vi "Add Modifier to File Name.vi"(1 "file name modifier":string, 2 "base path":path) -> (0 "appended path":path)   [LabVIEW 2021, in "Logging.lvlib"]
doc: "Take 'base path' and append 'file name modifier' to the name part of the path, keeping the same exension. Returned in 'appended path'."
uses:
  Logging.lvlib
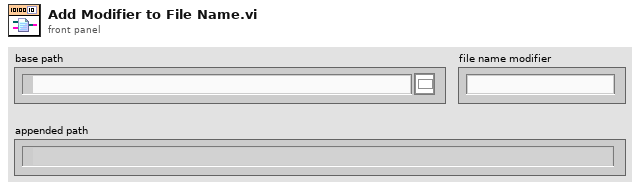
[diagram p1: front panel]
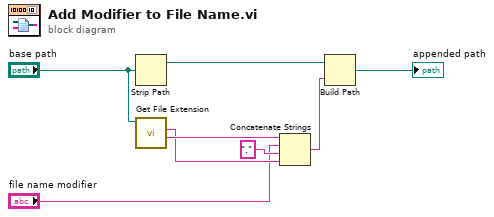
[diagram p0: block diagram]
diagram:
  n1 = Strip Path(path="base path") -> (stripped path=w5:path)  [unwired: 1 out]
  n2 = call <vilib>:"Get File Extension.vi"("file"="base path") -> ("filename without extension"=w6:string, "lowercase file extension"=w4:string)  [unwired: 6 in, 3 out]
  n3 = Concatenate Strings(w6, "file name modifier", "." ("string"), w4) -> (w7:string)
  n4 = Build Path(base path=w5, name or relative path=w7) -> (appended path=→"appended path":path)
